vi "Read Session.vi"(8 "error in (no error)":errorcluster, 11 "Camera Imaqdx CFG in":refnum<class "Camera Imaqdx CFG.lvclass">) -> (0 "error out":errorcluster, 2 "IMAQdx Session":T1, 3 "Camera Imaqdx CFG out":refnum<class "Camera Imaqdx CFG.lvclass">)   [LabVIEW 2023, in "HAL.lvlib" / "Camera Imaqdx CFG.lvclass"]
uses:
  Camera Imaqdx CFG.lvclass
  Camera Imaqdx CFG.lvclass/Camera Imaqdx CFG.ctl
  <vilib>/userDefined/High Color/IMAQdx.ctl
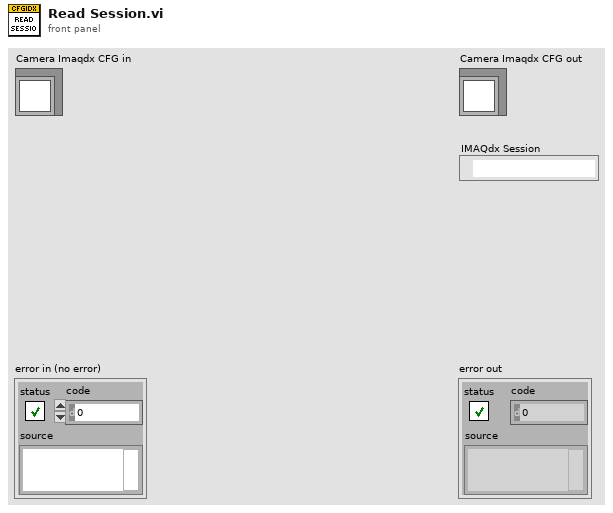
[diagram p1: front panel]
types:
  T1 = typedef "IMAQdx.ctl" = refnum<k21>
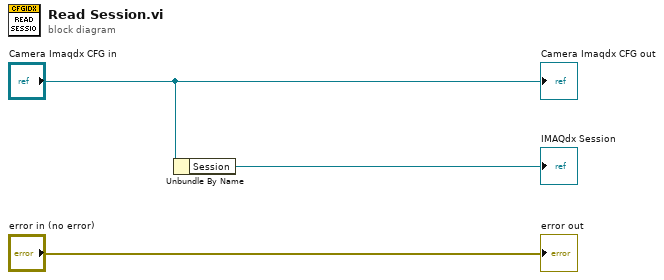
[diagram p0: block diagram]
diagram:
  n1 = Unbundle By Name("Camera Imaqdx CFG in") -> ("Session"=→"IMAQdx Session":T1)
  "error out" <- "error in (no error)"
  "Camera Imaqdx CFG out" <- "Camera Imaqdx CFG in"
